vi "Halverson_EMP_Fast.vi"(0 "tolerance":dbl=1e-13, 1 "Error Analysis":u16(ring)=4 items=["Max", "Max_Norm", "Norm", "Last Value", "Last Constant"], 3 "Шаг h, с":dbl=0.01, 4 "k":i32=4, 5 "Время, с":dbl=30.0, 7 "Hmax":dbl=1.0, 8 "Parameter":dbl[](array[numeric])=[1.4, 1.4, 1.4], 10 "last_point_Thomas":dbl[](array[numeric])=[2.3727475682665875, 0.23609824454436878, 0.4447912442126299], 13 "Hmin":dbl=0.001, 15 "Points count":i32=2, 18 "n":i32[](array[numeric])=[2, 4, 6, 8, 10, 12, 14, 16, 18, 20, 22], 19 "Ext.Type":u16(ring) items=["FNode", "MathScript", "ECD8 Arrays", "ECD8 Fnode", "ECD8 FnodeDiv", "FNode Exp"]) -> (6 "Elapsed Time":dbl=0.06815049055421696, 12 "Number of steps":i32=5381, 14 "Error Estimation":dbl=10.705281037182138, 17 "Rejected steps":i32=4)   [LabVIEW 2016]
uses:
  <vilib>/Analysis/_algsub.llb/Real Vector Norm.vi
  <vilib>/Analysis/5stat.llb/RMS (DBL).vi
  <vilib>/Analysis/NI_AALBase.lvlib
  <vilib>/Analysis/NI_AALPro.lvlib
panel:
  in  "Initial Conditions":dbl[](array[numeric])=[1.0, 0.0, 1.0]
  out "Last Value Reference":dbl[](array[numeric])=[-8.12716166984979, -1.7528766973053886, -0.13869544413081428] format="%#_15f"
  out "Rejected Steps":i32[](graph)
  out "Last Value":dbl[](array[numeric])=[-8.129137215287567, -1.7586488541882352, -0.13351843935062088] format="%#_15f"
  out "Step time variation":dbl[](graph)=[0.07219387728946458, 0.06410710381896934]
  out "Real Error":dbl[][](graph)
  out "Step Variation":dbl[](graph)
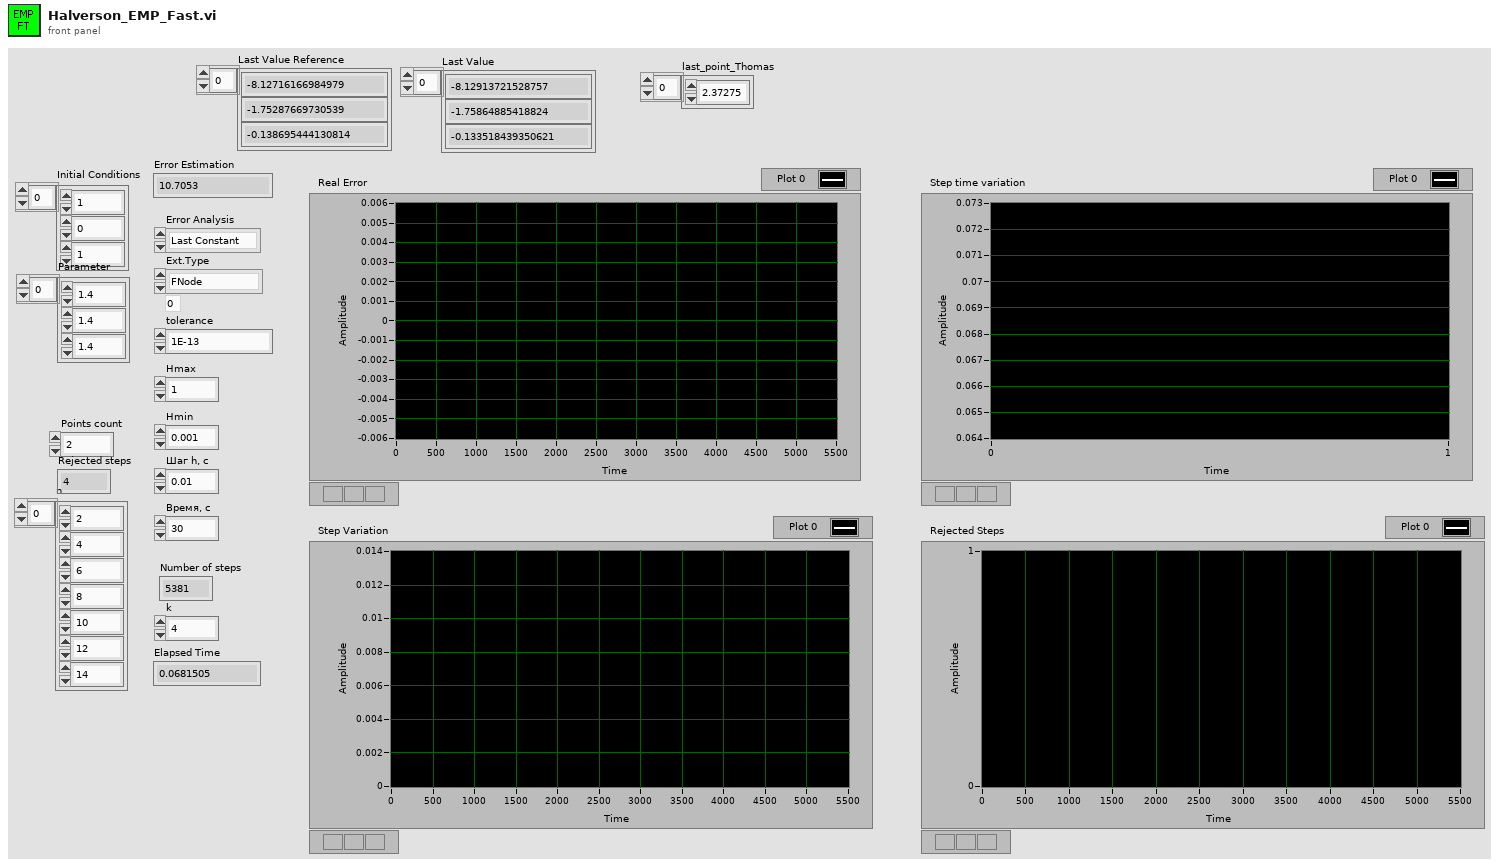
[diagram p1: front panel]
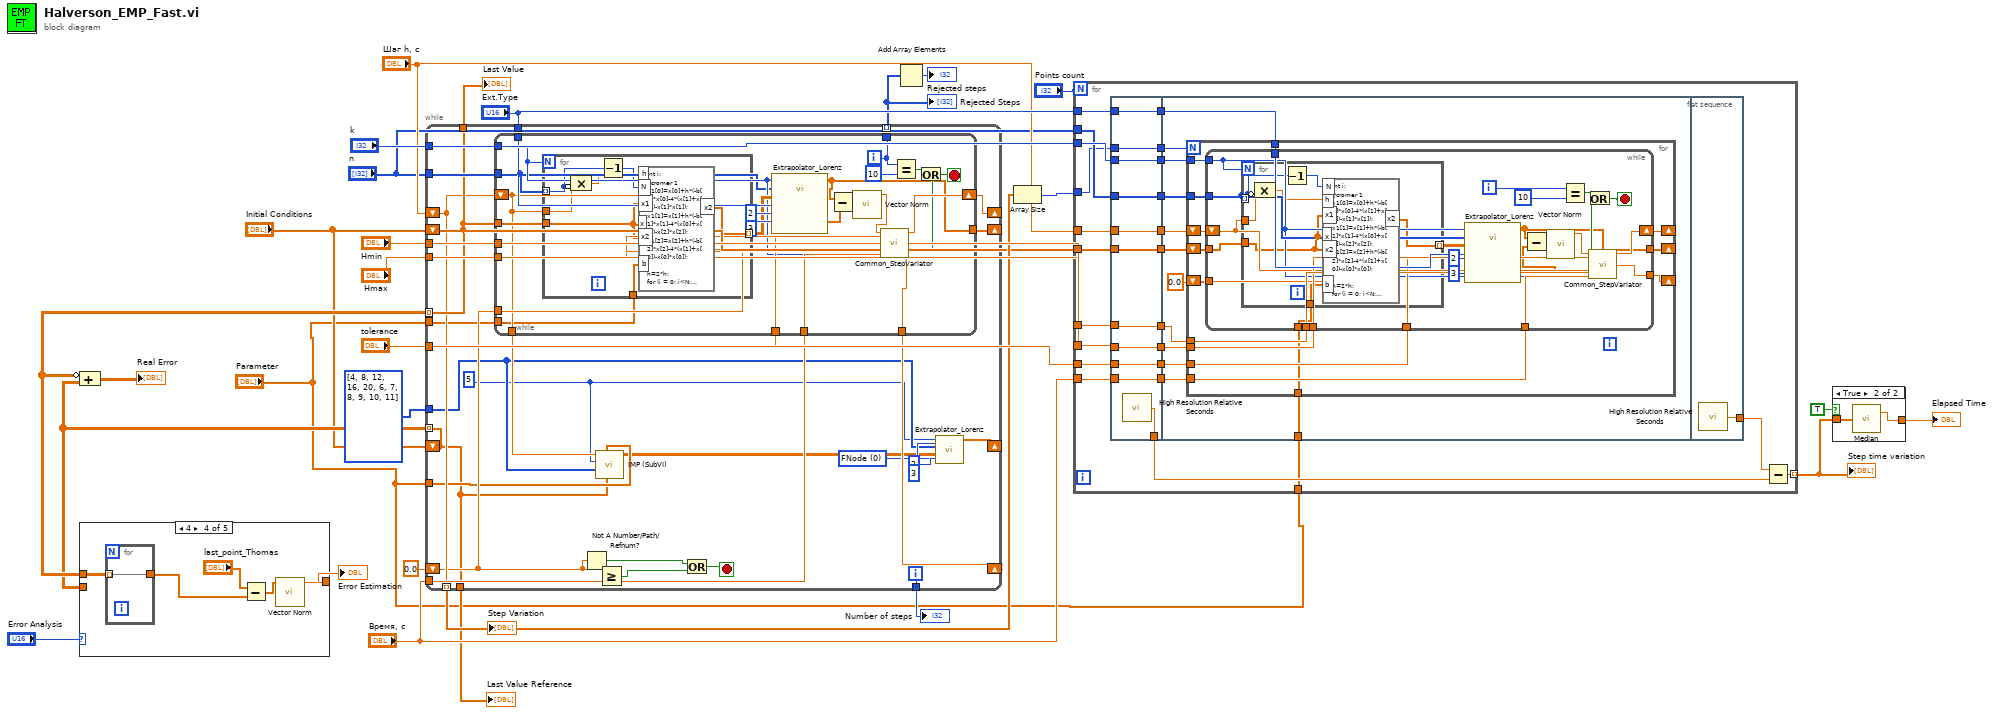
[diagram p0: block diagram]
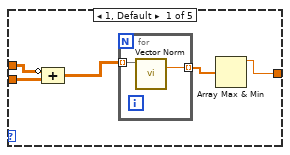
[diagram p2: hidden frame]
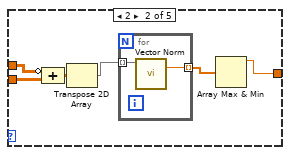
[diagram p3: hidden frame]
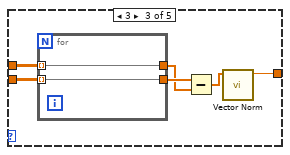
[diagram p4: hidden frame]
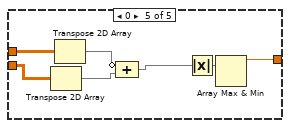
[diagram p5: hidden frame]
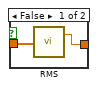
[diagram p6: hidden frame]
diagram:
  n1 = while {
    shift-right: [w50] -> _
    shift-left: "Initial Conditions" -> [w43]
    tunnel: "n" -> [w57]
    tunnel: "k" -> [w55]
    tunnel: "Ext.Type" -> [w46]
    shift-right: [w54] -> _
    shift-left: "Шаг h, с" -> [w37]
    shift-right: [w45] -> _
    shift-left: 0.0 -> [w36]
    tunnel: [w37] -> w13 mode=indexing
    tunnel: "Время, с" -> [w44]
    tunnel: [w56] -> w23
    tunnel: "tolerance" -> [w51]
    tunnel: "Hmin" -> [w53]
    tunnel: "Hmax" -> [w52]
    tunnel: [w43] -> w6 mode=indexing
    shift-right: [w49] -> _
    shift-left: "Initial Conditions" -> [w30]
    tunnel: i32[] [4, 8, 12, 16, 20, 6, 7, 8, 9, 10, 11] ("n 2") -> [w33]
    tunnel: [w30] -> w5 mode=indexing
    tunnel: [w43] -> w11
    tunnel: [w42] -> w10 mode=indexing
    tunnel: [w30] -> w4
    tunnel: "Parameter" -> [w31]
    tunnel: "Parameter" -> [w35]
    i -> [w56]
    stop <- w39 stop-if-true
    w41 = u16 0 items=["FNode", "MathScript", "ECD8 Arrays", "ECD8 Fnode", "ECD8 FnodeDiv"] ("Ext.Type")
    w32 = 5
    n2 = while {
      tunnel: w57 -> [w64]
      tunnel: w55 -> [w66]
      tunnel: w53 -> [w81]
      tunnel: w52 -> [w80]
      tunnel: w51 -> [w79]
      tunnel: [w60] -> w50
      tunnel: w46 -> [w76]
      tunnel: [w69] -> w45
      tunnel: w44 -> [w75]
      tunnel: w43 -> [w65]
      shift-right: [w82] -> w54
      shift-left: w37 -> [w63]
      tunnel: [w63] -> w34
      tunnel: [w70] -> w42
      tunnel: w36 -> [w68]
      tunnel: w35 -> [w62]
      i -> [w70]
      stop <- w72 stop-if-true
      n3 = for {
        N: w66 -> [_]
        tunnel: [w87] -> w67 mode=indexing
        tunnel: w64 -> [w88] mode=indexing
        tunnel: w63 -> [w89]
        tunnel: w65 -> [w85]
        tunnel: w62 -> [w83]
        n4 = Compound Arithmetic op=MULTIPLY(w89, invert w88) -> (w86:dbl)
        n5 = Decrement(x=w88) -> (x-1=w84:i32)
        n6 = formula code="int i;\n//cromer 1\nx1[0]=x[0]+h*(-b[0]*x[0]-4*(x[1]+x[2])-x[1]*x[1]);\nx1[1]=x[1]+h*(-b[1]*x[1]-4*(x[0]+x[2])-x[2]*x[2]);\nx1[2]=x[2]+h*(-b[2]*x[2]-4*(x[1]+x[0])-x[0]*x[0]);\n\nh=2*h;\nfor (i = 0; i<N; i++)\n{\n//EEuler\nx2[0]=x[0]+h*(-b[0]*x1[0]-4*(x1[1]+x1[2])-x1[1]*x1[1]);\nx2[1]=x[1]+h*(-b[1]*x1[1]-4*(x1[0]+x1[2])-x1[2]*x1[2]);\nx2[2]=x[2]+h*(-b[2]*x1[2]-4*(x1[1]+x1[0])-x1[0]*x1[0]);\n\nx[0]=x1[0];\nx[1]=x1[1];\nx[2]=x1[2];\nx1[0]=x2[0];\nx1[1]=x2[1];\nx1[2]=x2[2];\n};"("x"=w85, "x1"=w85, "h"=w86, "x2"=w85, "N"=w84, "b"=w83) -> ("x2"=w87:dbl[])
      }
      n7 = call "Extrapolator_Lorenz.vi"("Порядок экстраполятора"=2 ("input variable"), "Dimension"=3 ("input variable"), "Ext.Type"=w76, "Х - нач. условия"=w67, "n"=w64, "k"=w66) -> ("TPrev"=w59:dbl[], "Tout"=w60:dbl[])  [unwired: 4 in]
      n8 = Subtract(x=w60, y=w59) -> (x-y=w61:dbl[])
      n9 = call-poly <vilib>:"Vector Norm.vi"("Input Vector"=w61) -> ("norm"=w58:dbl)  [unwired: 9 in, 1 out]
      n10 = call "Common_StepVariator.vi"("err"=w58, "tolerance"=w79, "Hmax"=w80, "Шаг h, с"=w63, "Current time"=w68, "k"=w66, "Hmin"=w81, "tmax"=w75) -> ("Hnew"=w82:dbl, "New time"=w69:dbl, "stop"=w71:bool)  [unwired: 4 in, 1 out]
      n11 = Equal?(x=w70, y=10) -> (x = y?=w74:bool)
      n12 = Or(x=w74, y=w71) -> (x .or. y?=w72:bool)
    }
    n13 = Not A Number/Path/Refnum?(number/path/refnum=w36) -> (NaN/Path/Refnum?=w40:bool)
    n14 = call "IMP (SubVI).vi"("Initial Conditions in"=w30, "b"=w31, "n in"=w33, "Numeric"=w32, "Шаг h, с"=w34) -> ("Initial Conditions out"=w29:dbl[][])  [unwired: 6 in]
    n15 = Greater Or Equal?(x=w36, y=w44) -> (x >= y?=w38:bool)
    n16 = Or(x=w40, y=w38) -> (x .or. y?=w39:bool)
    n17 = call "Extrapolator_Lorenz.vi"("Порядок экстраполятора"=2, "Dimension"=3, "Ext.Type"=w41, "Х - нач. условия"=w29, "n"=w33, "k"=w32) -> ("Tout"=w49:dbl[])  [unwired: 4 in, 1 out]
  }
  "Step Variation" <- w13
  "Number of steps" <- w23
  "Last Value" <- w11
  "Rejected Steps" <- w10
  "Last Value Reference" <- w4
  n18 = Compound Arithmetic op=ADD(invert w6, w5) -> (→"Real Error":dbl[][])
  n19 = case shown="4" "Error Analysis" {
    tunnel: w5 -> [w91 w99 w108 _ w119]
    tunnel: [w93 w101 w110 w117 w124] -> w8
    tunnel: w6 -> [w92 w100 w109 w116 w120]
    frame 1, Default {
      n20 = Compound Arithmetic op=ADD(invert w92, w91) -> (w90:dbl[][])
      n21 = for {
        tunnel: [w96] -> w94 mode=indexing
        tunnel: w90 -> [w95] mode=indexing
        n22 = call-poly <vilib>:"Vector Norm.vi"("Input Vector"=w95) -> ("norm"=w96:dbl)  [unwired: 9 in, 1 out]
      }
      n23 = Array Max & Min(array=w94) -> (max value=w93:dbl)  [unwired: 3 out]
    }
    frame 2 {
      n24 = Compound Arithmetic op=ADD(invert w100, w99) -> (w98:dbl[][])
      n25 = Transpose 2D Array(2D array=w98) -> (transposed array=w97:dbl[][])
      n26 = for {
        tunnel: [w104] -> w102 mode=indexing
        tunnel: w97 -> [w103] mode=indexing
        n27 = call-poly <vilib>:"Vector Norm.vi"("Input Vector"=w103) -> ("norm"=w104:dbl)  [unwired: 9 in, 1 out]
      }
      n28 = Array Max & Min(array=w102) -> (max value=w101:dbl)  [unwired: 3 out]
    }
    frame 3 {
      n29 = for {
        tunnel: w109 -> [w112] mode=indexing
        tunnel: [w112] -> w106
        tunnel: w108 -> [w111] mode=indexing
        tunnel: [w111] -> w107
      }
      n30 = Subtract(x=w107, y=w106) -> (x-y=w105:dbl[])
      n31 = call-poly <vilib>:"Vector Norm.vi"("Input Vector"=w105) -> ("norm"=w110:dbl)  [unwired: 9 in, 1 out]
    }
    frame 4 {
      n32 = for {
        tunnel: w116 -> [w118] mode=indexing
        tunnel: [w118] -> w115
      }
      n33 = Subtract(x="last_point_Thomas", y=w115) -> (x-y=w114:dbl[])
      n34 = call-poly <vilib>:"Vector Norm.vi"("Input Vector"=w114) -> ("norm"=w117:dbl)  [unwired: 9 in, 1 out]
    }
    frame 0 {
      n35 = Transpose 2D Array(2D array=w119) -> (transposed array=w122:dbl[][])
      n36 = Transpose 2D Array(2D array=w120) -> (transposed array=w123:dbl[][])
      n37 = Compound Arithmetic op=ADD(invert w123, w122) -> (w121:dbl[][])
      n38 = Absolute Value(x=w121) -> (abs(x)=w125:dbl[][])
      n39 = Array Max & Min(array=w125) -> (max value=w124:dbl)  [unwired: 3 out]
    }
  }
  "Error Estimation" <- w8
  n40 = Add Array Elements(numeric array=w10) -> (sum=→"Rejected steps":i32)
  n41 = Array Size(array=w13) -> (size(s)=w22:i32)
  n42 = for {
    N: "Points count" -> [_]
    tunnel: "k" -> [w149]
    tunnel: "n" -> [w148]
    tunnel: "Ext.Type" -> [w128]
    tunnel: "Initial Conditions" -> [w147]
    tunnel: w22 -> [w146]
    tunnel: [w139] -> w20 mode=indexing
    tunnel: "Шаг h, с" -> [w130]
    tunnel: "Hmin" -> [w138]
    tunnel: "Hmax" -> [w135]
    tunnel: "tolerance" -> [w134]
    tunnel: "Время, с" -> [w132]
    tunnel: "Parameter" -> [w126]
    n43 = flat-sequence {
      tunnel: w146 -> [w157]
      tunnel: w147 -> [w158]
      tunnel: w148 -> [w159]
      tunnel: w149 -> [w160]
      tunnel: [w160] -> w145
      tunnel: [w159] -> w144
      tunnel: [w158] -> w143
      tunnel: [w157] -> w142
      tunnel: [w156] -> w140
      tunnel: w138 -> [w155]
      tunnel: [w155] -> w137
      tunnel: w135 -> [w154]
      tunnel: [w154] -> w136
      tunnel: w134 -> [w153]
      tunnel: [w153] -> w133
      tunnel: w132 -> [w152]
      tunnel: [w152] -> w131
      tunnel: w130 -> [w151]
      tunnel: [w151] -> w129
      tunnel: w128 -> [w150]
      tunnel: [w150] -> w127
      tunnel: w145 -> [w172]
      tunnel: w144 -> [w171]
      tunnel: w143 -> [w170]
      tunnel: w142 -> [w169]
      tunnel: w137 -> [w167]
      tunnel: w136 -> [w166]
      tunnel: w133 -> [w165]
      tunnel: w131 -> [w164]
      tunnel: w129 -> [w163]
      tunnel: w127 -> [w162]
      tunnel: w126 -> [w161]
      tunnel: [w219] -> w141
      frame #0 {
        n44 = call <vilib>:"High Resolution Relative Seconds.vi"() -> ("relative seconds"=w156:dbl)
      }
      frame #1 {
        n45 = for {
          N: w169 -> [_]
          shift-right: [w182] -> _
          shift-left: w170 -> [w184]
          tunnel: w171 -> [w186]
          tunnel: w172 -> [w181]
          tunnel: w162 -> [w185]
          shift-right: [w183] -> _
          shift-left: w163 -> [w176]
          tunnel: w167 -> [w180]
          tunnel: w166 -> [w179]
          tunnel: w165 -> [w178]
          shift-right: [w175] -> _
          shift-left: 0.0 -> [w174]
          tunnel: w164 -> [w177]
          tunnel: w161 -> [w173]
          n46 = while {
            tunnel: w186 -> [w194]
            tunnel: w185 -> [w211]
            tunnel: w184 -> [w195]
            tunnel: [w189] -> w182
            tunnel: w181 -> [w193]
            tunnel: w180 -> [w207]
            tunnel: w179 -> [w206]
            tunnel: w178 -> [w205]
            tunnel: w174 -> [w204]
            tunnel: w177 -> [w203]
            shift-right: [w208] -> w183
            shift-left: w176 -> [w196]
            tunnel: [w197] -> w175
            tunnel: w173 -> [w191]
            i -> [w199]
            stop <- w200 stop-if-true
            n47 = for {
              N: w193 -> [_]
              tunnel: w194 -> [w217] mode=indexing
              tunnel: w196 -> [w218]
              tunnel: w195 -> [w216]
              tunnel: [w213] -> w192 mode=indexing
              tunnel: w191 -> [w212]
              n48 = Compound Arithmetic op=MULTIPLY(w218, invert w217) -> (w214:dbl)
              n49 = Decrement(x=w217) -> (x-1=w215:i32)
              n50 = formula code="int i;\n//cromer 1\nx1[0]=x[0]+h*(-b[0]*x[0]-4*(x[1]+x[2])-x[1]*x[1]);\nx1[1]=x[1]+h*(-b[1]*x[1]-4*(x[0]+x[2])-x[2]*x[2]);\nx1[2]=x[2]+h*(-b[2]*x[2]-4*(x[1]+x[0])-x[0]*x[0]);\n\nh=2*h;\nfor (i = 0; i<N; i++)\n{\n//EEuler\nx2[0]=x[0]+h*(-b[0]*x1[0]-4*(x1[1]+x1[2])-x1[1]*x1[1]);\nx2[1]=x[1]+h*(-b[1]*x1[1]-4*(x1[0]+x1[2])-x1[2]*x1[2]);\nx2[2]=x[2]+h*(-b[2]*x1[2]-4*(x1[1]+x1[0])-x1[0]*x1[0]);\n\nx[0]=x1[0];\nx[1]=x1[1];\nx[2]=x1[2];\nx1[0]=x2[0];\nx1[1]=x2[1];\nx1[2]=x2[2];\n};"("x"=w216, "x1"=w216, "h"=w214, "x2"=w216, "N"=w215, "b"=w212) -> ("x2"=w213:dbl[])
            }
            n51 = call "Extrapolator_Lorenz.vi"("Порядок экстраполятора"=2 ("input variable"), "Dimension"=3 ("input variable"), "Ext.Type"=w211, "Х - нач. условия"=w192, "n"=w194, "k"=w193) -> ("TPrev"=w188:dbl[], "Tout"=w189:dbl[])  [unwired: 4 in]
            n52 = Subtract(x=w189, y=w188) -> (x-y=w190:dbl[])
            n53 = call-poly <vilib>:"Vector Norm.vi"("Input Vector"=w190) -> ("norm"=w187:dbl)  [unwired: 9 in, 1 out]
            n54 = Equal?(x=w199, y=10) -> (x = y?=w201:bool)
            n55 = call "Common_StepVariator.vi"("err"=w187, "tolerance"=w205, "Hmax"=w206, "Шаг h, с"=w196, "Current time"=w204, "k"=w193, "Hmin"=w207, "tmax"=w203) -> ("Hnew"=w208:dbl, "New time"=w197:dbl, "stop"=w198:bool)  [unwired: 4 in, 1 out]
            n56 = Or(x=w201, y=w198) -> (x .or. y?=w200:bool)
          }
        }
      }
      frame #2 {
        n57 = call <vilib>:"High Resolution Relative Seconds.vi"() -> ("relative seconds"=w219:dbl)
      }
    }
    n58 = Subtract(x=w141, y=w140) -> (x-y=w139:dbl)
  }
  "Step time variation" <- w20
  n59 = case shown="True" TRUE {
    tunnel: w20 -> [w220 w223]
    tunnel: [w221 w222] -> w19
    frame False {
      n60 = call-poly <vilib>:"RMS.vi"("X"=w220) -> ("rms value"=w221:dbl)  [unwired: 1 out]
    }
    frame True {
      n61 = call <vilib>:"Median.vi"("X"=w223) -> ("median"=w222:dbl)  [unwired: 1 out]
    }
  }
  "Elapsed Time" <- w19
